vi "VI_ScrollMCListboxDown.vi"(8 "error in (no error)":errorcluster, 11 "MCListbox ref":refnum<vi>) -> (0 "error out":errorcluster, 3 "MCListbox ref out":refnum<vi>)   [LabVIEW 2018]
uses:
  <vilib>/Utility/miscctls.llb/LVRowAndColumnUnsignedTypeDef.ctl
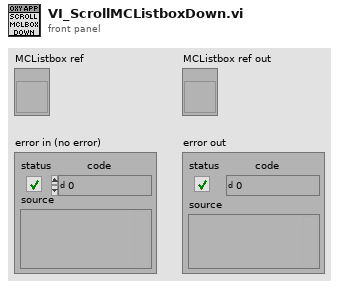
[diagram p1: front panel]
types:
  T1 = typedef "LVRowAndColumnUnsignedTypeDef.ctl" = cluster{"Row":u32, "Column":u32}
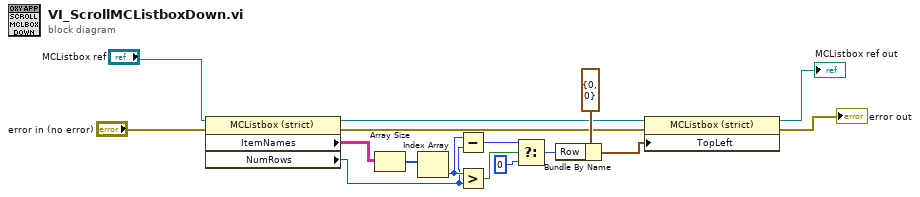
[diagram p0: block diagram]
diagram:
  n1 = property class="MCListbox (strict)"(reference="MCListbox ref", error in="error in (no error)") -> (reference out=w1:refnum<vi>, error out=w2:errorcluster, "ItemNames"=w9:string[][], "NumRows"=w8:u32)
  n2 = Array Size(array=w9) -> (size(s)=w16:i32[])
  n3 = Index Array(array=w16) -> (element=w13:i32)  [unwired: 1 in]
  n4 = Subtract(x=w13, y=w8) -> (x-y=w12:u32)
  n5 = Greater?(x=w13, y=w8) -> (0:w14:bool)
  n6 = Select(t=w12, s=w14, f=u32 0) -> (s? t:f=w10:u32)
  n7 = Bundle By Name(cluster=T1 {"Row"=0, "Column"=0} ("input cluster"), "Row"=w10) -> (w7:T1)
  n8 = property class="MCListbox (strict)"(reference=w1, error in=w2, "TopLeft"=w7) -> (reference out=→"MCListbox ref out":refnum<vi>, error out=→"error out":errorcluster)
